vi "uTTA_SetPreHeatingTime.vi"(4 "error in":errorcluster, 6 "PreHeatingTime (s)":u32, 7 "VISA Refnum in":refnum<visa-resource-name>) -> (0 "error out":errorcluster, 2 "Received":string, 3 "VISA Refnum out":refnum<visa-resource-name>)   [LabVIEW 2021]
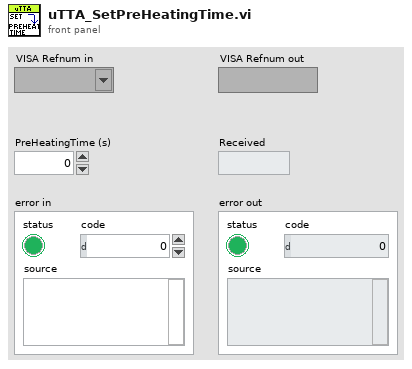
[diagram p1: front panel]
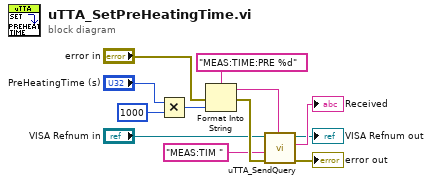
[diagram p0: block diagram]
diagram:
  n1 = Multiply(x="PreHeatingTime (s)", y=u32 1000) -> (x*y=w5:u32)
  n2 = Format Into String(format string="MEAS:TIME:PRE %d", error in="error in", w5) -> (resulting string=w9:string, error out=w11:errorcluster)  [unwired: 1 in]
  n3 = call "uTTA_SendQuery.vi"("Send String"=w9, "error in (no error)"=w11, "Response Qualifier(\"\")"="MEAS:TIM " ("Response Qualifier(\"\")"), "VISA Refnum in"="VISA Refnum in") -> ("error out"=→"error out":errorcluster, "Received"=→"Received":string, "VISA Refnum out"=→"VISA Refnum out":refnum<visa-resource-name>)  [unwired: 5 in]
